vi "Begin.vi"(8 "error in":errorcluster) -> (0 "error out":errorcluster)   [LabVIEW 2020]
doc: "Called before other user functions, this VI is expected to open initial I/O refnums, load in file data, and do all program initialization. Notice that the <B>error out</B> terminal is simply used for data flow. Wiring it to other structures or subVIs ensures that this VI runs first."
uses:
  <vilib>/Rock Robotics/WPI/ThirdParty/Phoenix-LabVIEW/Motor Controller/Controls/CTRE_Phoenix_MotorControl_TalonFXMotorControllerConfigurables.ctl
  <vilib>/Rock Robotics/WPI/ThirdParty/Phoenix-LabVIEW/Motor Controller/Controls/CTRE_Phoenix_MotorControl_BaseConfigurables.ctl
  <vilib>/Rock Robotics/WPI/ThirdParty/Phoenix-LabVIEW/Motor Controller/Controls/CTRE_Phoenix_MotorControl_VelocityMeasurementPeriod.ctl
  <vilib>/Rock Robotics/WPI/ThirdParty/Phoenix-LabVIEW/Motor Controller/Controls/CTRE_Phoenix_MotorControl_SlotStructure.ctl
  <vilib>/Rock Robotics/WPI/ThirdParty/Phoenix-LabVIEW/Motor Controller/Controls/CTRE_Phoenix_MotorControl_FilterStruct.ctl
  <vilib>/Rock Robotics/WPI/ThirdParty/Phoenix-LabVIEW/Motor Controller/Controls/CTRE_Phoenix_MotorControl_RemoteSourceType.ctl
  <vilib>/Rock Robotics/WPI/ThirdParty/Phoenix-LabVIEW/Controls/CTRE_Phoenix_CustomParamConfiguration.ctl
  <vilib>/Rock Robotics/WPI/ThirdParty/Phoenix-LabVIEW/Motor Controller/Controls/CTRE_Phoenix_MotorControl_FeedbackDevice_TalonFX.ctl
  <vilib>/Rock Robotics/WPI/ThirdParty/Phoenix-LabVIEW/Motor Controller/Controls/CTRE_Phoenix_MotorControl_LimitSwitchNormal.ctl
  <vilib>/Rock Robotics/WPI/ThirdParty/Phoenix-LabVIEW/Motor Controller/Controls/CTRE_Phoenix_MotorControl_LimitSwitchSource_Local.ctl
  <vilib>/Rock Robotics/WPI/ThirdParty/Phoenix-LabVIEW/Motor Controller/Controls/CTRE_Phoenix_MotorControl_SupplyCurrentLimitConfiguration.ctl
  <vilib>/Rock Robotics/WPI/ThirdParty/Phoenix-LabVIEW/Motor Controller/Controls/CTRE_Phoenix_MotorControl_StatorCurrentLimitConfiguration.ctl
  <vilib>/Rock Robotics/WPI/ThirdParty/Phoenix-LabVIEW/Motor Controller/Controls/CTRE_Phoenix_MotorControl_MotorCommutation_TalonFX.ctl
  <vilib>/Rock Robotics/WPI/ThirdParty/Phoenix-LabVIEW/CANCoder/Controls/CTRE_Phoenix_CANcoder_AbsoluteSensorRange.ctl
  <vilib>/Rock Robotics/WPI/ThirdParty/Phoenix-LabVIEW/CANCoder/Controls/CTRE_Phoenix_CANcoder_SensorInitializationStrategy.ctl
  <vilib>/Rock Robotics/WPI/ThirdParty/Phoenix-LabVIEW/Motor Controller/Controls/CTRE_Phoenix_MotorControl_NeutralMode.ctl
  <vilib>/Rock Robotics/SystemInterfaces/DIO/FPGA_DIOChannel.ctl
  <vilib>/Rock Robotics/WPI/DriverStation/WPI_DriverStationRobotMode2.ctl
  <vilib>/Rock Robotics/WPI/SafetyOutput/WPI_SafetyOutputConfigMenu.ctl
  <vilib>/Rock Robotics/WPI/RobotDrive/WPI_RobotDriveDevRef.ctl
  <vilib>/Rock Robotics/WPI/MotorControl/WPI_MotorControlDeviceRef.ctl
  <vilib>/Rock Robotics/WPI/MotorControl/WPI_MotorControlType.ctl
  <vilib>/Rock Robotics/SystemInterfaces/DIO/FPGA_DIOPWMChannel.ctl
  <vilib>/Rock Robotics/WPI/PWM/WPI_PWMDeadband.ctl
  <vilib>/Rock Robotics/WPI/ThirdParty/REV Robotics/REVLib/Typedef/Spark MAX Motor Type.ctl
  <vilib>/Rock Robotics/WPI/ThirdParty/REV Robotics/REVLib/Typedef/Spark MAX Idle Mode.ctl
  <vilib>/Rock Robotics/WPI/Joystick/WPI_JoystickDeviceEnum.ctl
  <vilib>/Rock Robotics/Network Tables/NT Write String Array.vi
  Robot Global Data.vi
  <vilib>/Rock Robotics/Network Tables/NT Write Boolean.vi
  <vilib>/Rock Robotics/WPI/Switch/WPI_SwitchOpenCounting.vi
  <vilib>/Rock Robotics/WPI/RobotDrive/WPI_RobotDriveOpen2MotorWithExistingMotors.vi
panel:
  in  "Tab Control":enum32{"DRIVE", "CLIMBING", "SHOOTER"}(tab)=enum."CLIMBING"
  in  "FALCON 500 DRIVE config":T1={"Base Configurables"={"openLoopRamp"=0.0, "closedLoopRamp"=0.0, "peakOutputForward"=1.0, "peakOutputReverse"=-1.0, "nominalOutputForward"=0.0, "nominalOutputReverse"=0.0, "neutralDeadband"=0.04, "voltageCompSaturation"=0.0, "voltageMeasurementFilter"=32, "velocityMeasurementPeriod"=100, "velocityMeasurementWindow"=64, "forwardSoftLimitThreshold"=0, "reverseSoftLimitThreshold"=0, "forwardSoftLimitEnable"=FALSE, "reverseSoftLimitEnable"=FALSE, "slot0"={"P"=0.0, "I"=0.0, "D"=0.0, "F"=0.0, "integralZone"=0.0, "allowableClosedLoopError"=0, "maxIntegralAccumulator"=0.0, "closedLoopPeakOutput"=1.0, "closedLoopPeriod"=1}, "slot1"={"P"=0.0, "I"=0.0, "D"=0.0, "F"=0.0, "integralZone"=0.0, "allowableClosedLoopError"=0, "maxIntegralAccumulator"=0.0, "closedLoopPeakOutput"=1.0, "closedLoopPeriod"=1}, "slot2"={"P"=0.0, "I"=0.0, "D"=0.0, "F"=0.0, "integralZone"=0.0, "allowableClosedLoopError"=0, "maxIntegralAccumulator"=0.0, "closedLoopPeakOutput"=1.0, "closedLoopPeriod"=1}, "slot3"={"P"=0.0, "I"=0.0, "D"=0.0, "F"=0.0, "integralZone"=0.0, "allowableClosedLoopError"=0, "maxIntegralAccumulator"=0.0, "closedLoopPeakOutput"=1.0, "closedLoopPeriod"=1}, "auxPIDPolarity"=FALSE, "remoteFilter0"={"remoteSensorDeviceID"=0, "remoteSensorSource"=enum."Off"}, "remoteFilter1"={"remoteSensorDeviceID"=0, "remoteSensorSource"=enum."Off"}, "motionCruiseVelocity"=0, "motionAcceleration"=0, "motionProfileTrajectoryPeriod"=0, "feedbackNotContinuous"=FALSE, "remoteSensorClosedLoopDisableNeutralOnLOS"=FALSE, "clearPositionOnLimitF"=FALSE, "clearPositionOnLimitR"=FALSE, "clearPositionOnQuadIdx"=FALSE, "limitSwitchDisableNeutralOnLOS"=FALSE, "softLimitDisableNeutralOnLOS"=FALSE, "pulseWidthPeriod_EdgesPerRot"=1, "pulseWidthPeriod_FilterWindowSz"=1, "customParam"={"customParam0"=0, "customParam1"=0}, "trajectoryInterpolationEnable"=TRUE}, "primaryPID"={"selectedFeedbackCoefficient"=1.0, "selectedFeedbackSensor"=1}, "auxiliaryPID"={"selectedFeedbackCoefficient"=1.0, "selectedFeedbackSensor"=1}, "forwardLimitSwitchNormal"=enum."Normally Open", "reverseLimitSwitchNormal"=enum."Normally Open", "forwardLimitSwitchDeviceID"=0, "reverseLimitSwitchDeviceID"=0, "forwardLimitSwitchSource"=enum."Feedback Connector", "reverseLimitSwitchSource"=enum."Feedback Connector", "sum0Term"=1, "sum1Term"=1, "diff0Term"=1, "diff1Term"=1, "Supply Current Limit Configuration"={"Enable?"=FALSE, "Current Limit"=0.0, "Threshold Current"=0.0, "Threshold Time"=0.0}, "Stator Current Limit Configuration"={"Enable?"=FALSE, "Current Limit"=0.0, "Threshold Current"=0.0, "Threshold Time"=0.0}, "Motor Commutation"=enum."Trapezoidal", "Absolute Sensor Range"=enum."Unsigned [0 to 360)", "Integrated Sensor Offset (Degrees)"=0.0, "Sensor Initialization Strategy"=enum."Boot To Zero"} {"diff1Term" items=["Integrated Sensor"=1, "Sensor Sum (S0 + S1)"=9, "Sensor Difference (D0 - D1)"=10, "Remote Source 0"=11, "Remote Source 1"=12, "None"=14, "Software Emulated"=15]; "diff0Term" items=["Integrated Sensor"=1, "Sensor Sum (S0 + S1)"=9, "Sensor Difference (D0 - D1)"=10, "Remote Source 0"=11, "Remote Source 1"=12, "None"=14, "Software Emulated"=15]; "sum1Term" items=["Integrated Sensor"=1, "Sensor Sum (S0 + S1)"=9, "Sensor Difference (D0 - D1)"=10, "Remote Source 0"=11, "Remote Source 1"=12, "None"=14, "Software Emulated"=15]; "sum0Term" items=["Integrated Sensor"=1, "Sensor Sum (S0 + S1)"=9, "Sensor Difference (D0 - D1)"=10, "Remote Source 0"=11, "Remote Source 1"=12, "None"=14, "Software Emulated"=15]; "auxiliaryPID"."selectedFeedbackSensor" items=["Integrated Sensor"=1, "Sensor Sum (S0 + S1)"=9, "Sensor Difference (D0 - D1)"=10, "Remote Source 0"=11, "Remote Source 1"=12, "None"=14, "Software Emulated"=15]; "primaryPID"."selectedFeedbackSensor" items=["Integrated Sensor"=1, "Sensor Sum (S0 + S1)"=9, "Sensor Difference (D0 - D1)"=10, "Remote Source 0"=11, "Remote Source 1"=12, "None"=14, "Software Emulated"=15]; "Base Configurables"."velocityMeasurementPeriod" items=["Period_1ms"=1, "Period_2ms"=2, "Period_5ms"=5, "Period_10ms"=10, "Period_20ms"=20, "Period_25ms"=25, "Period_50ms"=50, "Period_100ms"=100]}
  in  "drive wheel diameter (in)":dbl format="%.3g"
  in  "drive gearbox ratio":dbl
  out "wheel circumference":dbl
  in  "MASTER LEFT DRIVE CAN ID":u8=2
  in  "FALCON Climbing config":T1={"Base Configurables"={"openLoopRamp"=0.0, "closedLoopRamp"=0.0, "peakOutputForward"=1.0, "peakOutputReverse"=-1.0, "nominalOutputForward"=0.0, "nominalOutputReverse"=0.0, "neutralDeadband"=0.04, "voltageCompSaturation"=0.0, "voltageMeasurementFilter"=32, "velocityMeasurementPeriod"=100, "velocityMeasurementWindow"=64, "forwardSoftLimitThreshold"=0, "reverseSoftLimitThreshold"=0, "forwardSoftLimitEnable"=FALSE, "reverseSoftLimitEnable"=FALSE, "slot0"={"P"=0.0, "I"=0.0, "D"=0.0, "F"=0.0, "integralZone"=0.0, "allowableClosedLoopError"=0, "maxIntegralAccumulator"=0.0, "closedLoopPeakOutput"=1.0, "closedLoopPeriod"=1}, "slot1"={"P"=0.0, "I"=0.0, "D"=0.0, "F"=0.0, "integralZone"=0.0, "allowableClosedLoopError"=0, "maxIntegralAccumulator"=0.0, "closedLoopPeakOutput"=1.0, "closedLoopPeriod"=1}, "slot2"={"P"=0.0, "I"=0.0, "D"=0.0, "F"=0.0, "integralZone"=0.0, "allowableClosedLoopError"=0, "maxIntegralAccumulator"=0.0, "closedLoopPeakOutput"=1.0, "closedLoopPeriod"=1}, "slot3"={"P"=0.0, "I"=0.0, "D"=0.0, "F"=0.0, "integralZone"=0.0, "allowableClosedLoopError"=0, "maxIntegralAccumulator"=0.0, "closedLoopPeakOutput"=1.0, "closedLoopPeriod"=1}, "auxPIDPolarity"=FALSE, "remoteFilter0"={"remoteSensorDeviceID"=0, "remoteSensorSource"=enum."Off"}, "remoteFilter1"={"remoteSensorDeviceID"=0, "remoteSensorSource"=enum."Off"}, "motionCruiseVelocity"=0, "motionAcceleration"=0, "motionProfileTrajectoryPeriod"=0, "feedbackNotContinuous"=FALSE, "remoteSensorClosedLoopDisableNeutralOnLOS"=FALSE, "clearPositionOnLimitF"=FALSE, "clearPositionOnLimitR"=FALSE, "clearPositionOnQuadIdx"=FALSE, "limitSwitchDisableNeutralOnLOS"=FALSE, "softLimitDisableNeutralOnLOS"=FALSE, "pulseWidthPeriod_EdgesPerRot"=1, "pulseWidthPeriod_FilterWindowSz"=1, "customParam"={"customParam0"=0, "customParam1"=0}, "trajectoryInterpolationEnable"=TRUE}, "primaryPID"={"selectedFeedbackCoefficient"=1.0, "selectedFeedbackSensor"=1}, "auxiliaryPID"={"selectedFeedbackCoefficient"=1.0, "selectedFeedbackSensor"=1}, "forwardLimitSwitchNormal"=enum."Normally Open", "reverseLimitSwitchNormal"=enum."Normally Open", "forwardLimitSwitchDeviceID"=0, "reverseLimitSwitchDeviceID"=0, "forwardLimitSwitchSource"=enum."Feedback Connector", "reverseLimitSwitchSource"=enum."Feedback Connector", "sum0Term"=1, "sum1Term"=1, "diff0Term"=1, "diff1Term"=1, "Supply Current Limit Configuration"={"Enable?"=FALSE, "Current Limit"=0.0, "Threshold Current"=0.0, "Threshold Time"=0.0}, "Stator Current Limit Configuration"={"Enable?"=FALSE, "Current Limit"=0.0, "Threshold Current"=0.0, "Threshold Time"=0.0}, "Motor Commutation"=enum."Trapezoidal", "Absolute Sensor Range"=enum."Unsigned [0 to 360)", "Integrated Sensor Offset (Degrees)"=0.0, "Sensor Initialization Strategy"=enum."Boot To Zero"} {"diff1Term" items=["Integrated Sensor"=1, "Sensor Sum (S0 + S1)"=9, "Sensor Difference (D0 - D1)"=10, "Remote Source 0"=11, "Remote Source 1"=12, "None"=14, "Software Emulated"=15]; "diff0Term" items=["Integrated Sensor"=1, "Sensor Sum (S0 + S1)"=9, "Sensor Difference (D0 - D1)"=10, "Remote Source 0"=11, "Remote Source 1"=12, "None"=14, "Software Emulated"=15]; "sum1Term" items=["Integrated Sensor"=1, "Sensor Sum (S0 + S1)"=9, "Sensor Difference (D0 - D1)"=10, "Remote Source 0"=11, "Remote Source 1"=12, "None"=14, "Software Emulated"=15]; "sum0Term" items=["Integrated Sensor"=1, "Sensor Sum (S0 + S1)"=9, "Sensor Difference (D0 - D1)"=10, "Remote Source 0"=11, "Remote Source 1"=12, "None"=14, "Software Emulated"=15]; "auxiliaryPID"."selectedFeedbackSensor" items=["Integrated Sensor"=1, "Sensor Sum (S0 + S1)"=9, "Sensor Difference (D0 - D1)"=10, "Remote Source 0"=11, "Remote Source 1"=12, "None"=14, "Software Emulated"=15]; "primaryPID"."selectedFeedbackSensor" items=["Integrated Sensor"=1, "Sensor Sum (S0 + S1)"=9, "Sensor Difference (D0 - D1)"=10, "Remote Source 0"=11, "Remote Source 1"=12, "None"=14, "Software Emulated"=15]; "Base Configurables"."velocityMeasurementPeriod" items=["Period_1ms"=1, "Period_2ms"=2, "Period_5ms"=5, "Period_10ms"=10, "Period_20ms"=20, "Period_25ms"=25, "Period_50ms"=50, "Period_100ms"=100]}
  in  "Motor Control Neutral Mode":T16=enum."Override to Brake"
  in  "CLIMBER LEFT CAN ID":u8=6
  in  "ARM LEFT CAN ID":u8=11
  in  "CLIMBER RIGHT CAN ID":u8=7
  in  "ARM RIGHT CAN ID":u8=15
  in  "FALCON shooter config":T1={"Base Configurables"={"openLoopRamp"=0.0, "closedLoopRamp"=0.0, "peakOutputForward"=1.0, "peakOutputReverse"=-1.0, "nominalOutputForward"=0.0, "nominalOutputReverse"=0.0, "neutralDeadband"=0.04, "voltageCompSaturation"=0.0, "voltageMeasurementFilter"=32, "velocityMeasurementPeriod"=100, "velocityMeasurementWindow"=64, "forwardSoftLimitThreshold"=0, "reverseSoftLimitThreshold"=0, "forwardSoftLimitEnable"=FALSE, "reverseSoftLimitEnable"=FALSE, "slot0"={"P"=0.0, "I"=0.0, "D"=0.0, "F"=0.0, "integralZone"=0.0, "allowableClosedLoopError"=0, "maxIntegralAccumulator"=0.0, "closedLoopPeakOutput"=1.0, "closedLoopPeriod"=1}, "slot1"={"P"=0.0, "I"=0.0, "D"=0.0, "F"=0.0, "integralZone"=0.0, "allowableClosedLoopError"=0, "maxIntegralAccumulator"=0.0, "closedLoopPeakOutput"=1.0, "closedLoopPeriod"=1}, "slot2"={"P"=0.0, "I"=0.0, "D"=0.0, "F"=0.0, "integralZone"=0.0, "allowableClosedLoopError"=0, "maxIntegralAccumulator"=0.0, "closedLoopPeakOutput"=1.0, "closedLoopPeriod"=1}, "slot3"={"P"=0.0, "I"=0.0, "D"=0.0, "F"=0.0, "integralZone"=0.0, "allowableClosedLoopError"=0, "maxIntegralAccumulator"=0.0, "closedLoopPeakOutput"=1.0, "closedLoopPeriod"=1}, "auxPIDPolarity"=FALSE, "remoteFilter0"={"remoteSensorDeviceID"=0, "remoteSensorSource"=enum."Off"}, "remoteFilter1"={"remoteSensorDeviceID"=0, "remoteSensorSource"=enum."Off"}, "motionCruiseVelocity"=0, "motionAcceleration"=0, "motionProfileTrajectoryPeriod"=0, "feedbackNotContinuous"=FALSE, "remoteSensorClosedLoopDisableNeutralOnLOS"=FALSE, "clearPositionOnLimitF"=FALSE, "clearPositionOnLimitR"=FALSE, "clearPositionOnQuadIdx"=FALSE, "limitSwitchDisableNeutralOnLOS"=FALSE, "softLimitDisableNeutralOnLOS"=FALSE, "pulseWidthPeriod_EdgesPerRot"=1, "pulseWidthPeriod_FilterWindowSz"=1, "customParam"={"customParam0"=0, "customParam1"=0}, "trajectoryInterpolationEnable"=TRUE}, "primaryPID"={"selectedFeedbackCoefficient"=1.0, "selectedFeedbackSensor"=1}, "auxiliaryPID"={"selectedFeedbackCoefficient"=1.0, "selectedFeedbackSensor"=1}, "forwardLimitSwitchNormal"=enum."Normally Open", "reverseLimitSwitchNormal"=enum."Normally Open", "forwardLimitSwitchDeviceID"=0, "reverseLimitSwitchDeviceID"=0, "forwardLimitSwitchSource"=enum."Feedback Connector", "reverseLimitSwitchSource"=enum."Feedback Connector", "sum0Term"=1, "sum1Term"=1, "diff0Term"=1, "diff1Term"=1, "Supply Current Limit Configuration"={"Enable?"=FALSE, "Current Limit"=0.0, "Threshold Current"=0.0, "Threshold Time"=0.0}, "Stator Current Limit Configuration"={"Enable?"=FALSE, "Current Limit"=0.0, "Threshold Current"=0.0, "Threshold Time"=0.0}, "Motor Commutation"=enum."Trapezoidal", "Absolute Sensor Range"=enum."Unsigned [0 to 360)", "Integrated Sensor Offset (Degrees)"=0.0, "Sensor Initialization Strategy"=enum."Boot To Zero"} {"diff1Term" items=["Integrated Sensor"=1, "Sensor Sum (S0 + S1)"=9, "Sensor Difference (D0 - D1)"=10, "Remote Source 0"=11, "Remote Source 1"=12, "None"=14, "Software Emulated"=15]; "diff0Term" items=["Integrated Sensor"=1, "Sensor Sum (S0 + S1)"=9, "Sensor Difference (D0 - D1)"=10, "Remote Source 0"=11, "Remote Source 1"=12, "None"=14, "Software Emulated"=15]; "sum1Term" items=["Integrated Sensor"=1, "Sensor Sum (S0 + S1)"=9, "Sensor Difference (D0 - D1)"=10, "Remote Source 0"=11, "Remote Source 1"=12, "None"=14, "Software Emulated"=15]; "sum0Term" items=["Integrated Sensor"=1, "Sensor Sum (S0 + S1)"=9, "Sensor Difference (D0 - D1)"=10, "Remote Source 0"=11, "Remote Source 1"=12, "None"=14, "Software Emulated"=15]; "auxiliaryPID"."selectedFeedbackSensor" items=["Integrated Sensor"=1, "Sensor Sum (S0 + S1)"=9, "Sensor Difference (D0 - D1)"=10, "Remote Source 0"=11, "Remote Source 1"=12, "None"=14, "Software Emulated"=15]; "primaryPID"."selectedFeedbackSensor" items=["Integrated Sensor"=1, "Sensor Sum (S0 + S1)"=9, "Sensor Difference (D0 - D1)"=10, "Remote Source 0"=11, "Remote Source 1"=12, "None"=14, "Software Emulated"=15]; "Base Configurables"."velocityMeasurementPeriod" items=["Period_1ms"=1, "Period_2ms"=2, "Period_5ms"=5, "Period_10ms"=10, "Period_20ms"=20, "Period_25ms"=25, "Period_50ms"=50, "Period_100ms"=100]}
  in  "Motor Control Neutral Mode 2":T16=enum."Override to Brake"
  in  "SHOOTER CAN ID":u8=8
  in  "KICKER CAN ID":u8=10
  in  "KICKER COUNT DIO":T17
  # "Sum and Diff terms are ways to select more than one sensor as a feedback device. \n Sum 0 is the first feedback device to be used for the Sum term.\n Sum 1 is the feedback device to be added to Sum 0 for the Sum term.\n Diff 0 and Diff 1 work in a similar manner."
  # "These are only applicable\nif using a remote limit switch.\n\nLocal limit switches/no limit\nswitches do not use this."
  # "Current is below Current Limit AND\n\n(Requested output is weaker** than applied motor\noutput OR is in the opposite direction).\n/\nMotor output is set to requested output."
  # "Current is above Threshold Current for Threshold Time\n/\nReduce motor output (towards neutral)."
  # "Current is below Current Limit.\n/\nRamp motor output towards requested output."
  # "Current is above Current Limit.\n/\nReduce motor output (towards neutral)."
  # "*If the configured Peak Threshold is less than the Continuous Threshold, the applied Peak Threshold is set equal to the Configured Continuous Threshold in firmware.\n** Both requested output and applied motor output are in the same direction, and requested output is closer to neutral."
  # "False: Primary Output = PID[0] + PID[1]  ---  Auxiliary Output = PID[0] - PID[1]\nTrue:  Primary Output = PID[0] - PID[1] --- Auxiliary Output = PID[0] + PID[1]"
  # "Enable the motion profile executor to perform linear interpolation between profile points.  Defaults to True."
  # "Sum and Diff terms are ways to select more than one sensor as a feedback device. \n Sum 0 is the first feedback device to be used for the Sum term.\n Sum 1 is the feedback device to be added to Sum 0 for the Sum term.\n Diff 0 and Diff 1 work in a similar manner."
  # "These are only applicable\nif using a remote limit switch.\n\nLocal limit switches/no limit\nswitches do not use this."
  # "Current is below Current Limit AND\n\n(Requested output is weaker** than applied motor\noutput OR is in the opposite direction).\n/\nMotor output is set to requested output."
  # "Current is above Threshold Current for Threshold Time\n/\nReduce motor output (towards neutral)."
  # "Current is below Current Limit.\n/\nRamp motor output towards requested output."
  # "Current is above Current Limit.\n/\nReduce motor output (towards neutral)."
  # "*If the configured Peak Threshold is less than the Continuous Threshold, the applied Peak Threshold is set equal to the Configured Continuous Threshold in firmware.\n** Both requested output and applied motor output are in the same direction, and requested output is closer to neutral."
  # "False: Primary Output = PID[0] + PID[1]  ---  Auxiliary Output = PID[0] - PID[1]\nTrue:  Primary Output = PID[0] - PID[1] --- Auxiliary Output = PID[0] + PID[1]"
  # "Enable the motion profile executor to perform linear interpolation between profile points.  Defaults to True."
  # "Sum and Diff terms are ways to select more than one sensor as a feedback device. \n Sum 0 is the first feedback device to be used for the Sum term.\n Sum 1 is the feedback device to be added to Sum 0 for the Sum term.\n Diff 0 and Diff 1 work in a similar manner."
  # "These are only applicable\nif using a remote limit switch.\n\nLocal limit switches/no limit\nswitches do not use this."
  # "Current is below Current Limit AND\n\n(Requested output is weaker** than applied motor\noutput OR is in the opposite direction).\n/\nMotor output is set to requested output."
  # "Current is above Threshold Current for Threshold Time\n/\nReduce motor output (towards neutral)."
  # "Current is below Current Limit.\n/\nRamp motor output towards requested output."
  # "Current is above Current Limit.\n/\nReduce motor output (towards neutral)."
  # "*If the configured Peak Threshold is less than the Continuous Threshold, the applied Peak Threshold is set equal to the Configured Continuous Threshold in firmware.\n** Both requested output and applied motor output are in the same direction, and requested output is closer to neutral."
  # "False: Primary Output = PID[0] + PID[1]  ---  Auxiliary Output = PID[0] - PID[1]\nTrue:  Primary Output = PID[0] - PID[1] --- Auxiliary Output = PID[0] + PID[1]"
  # "Enable the motion profile executor to perform linear interpolation between profile points.  Defaults to True."
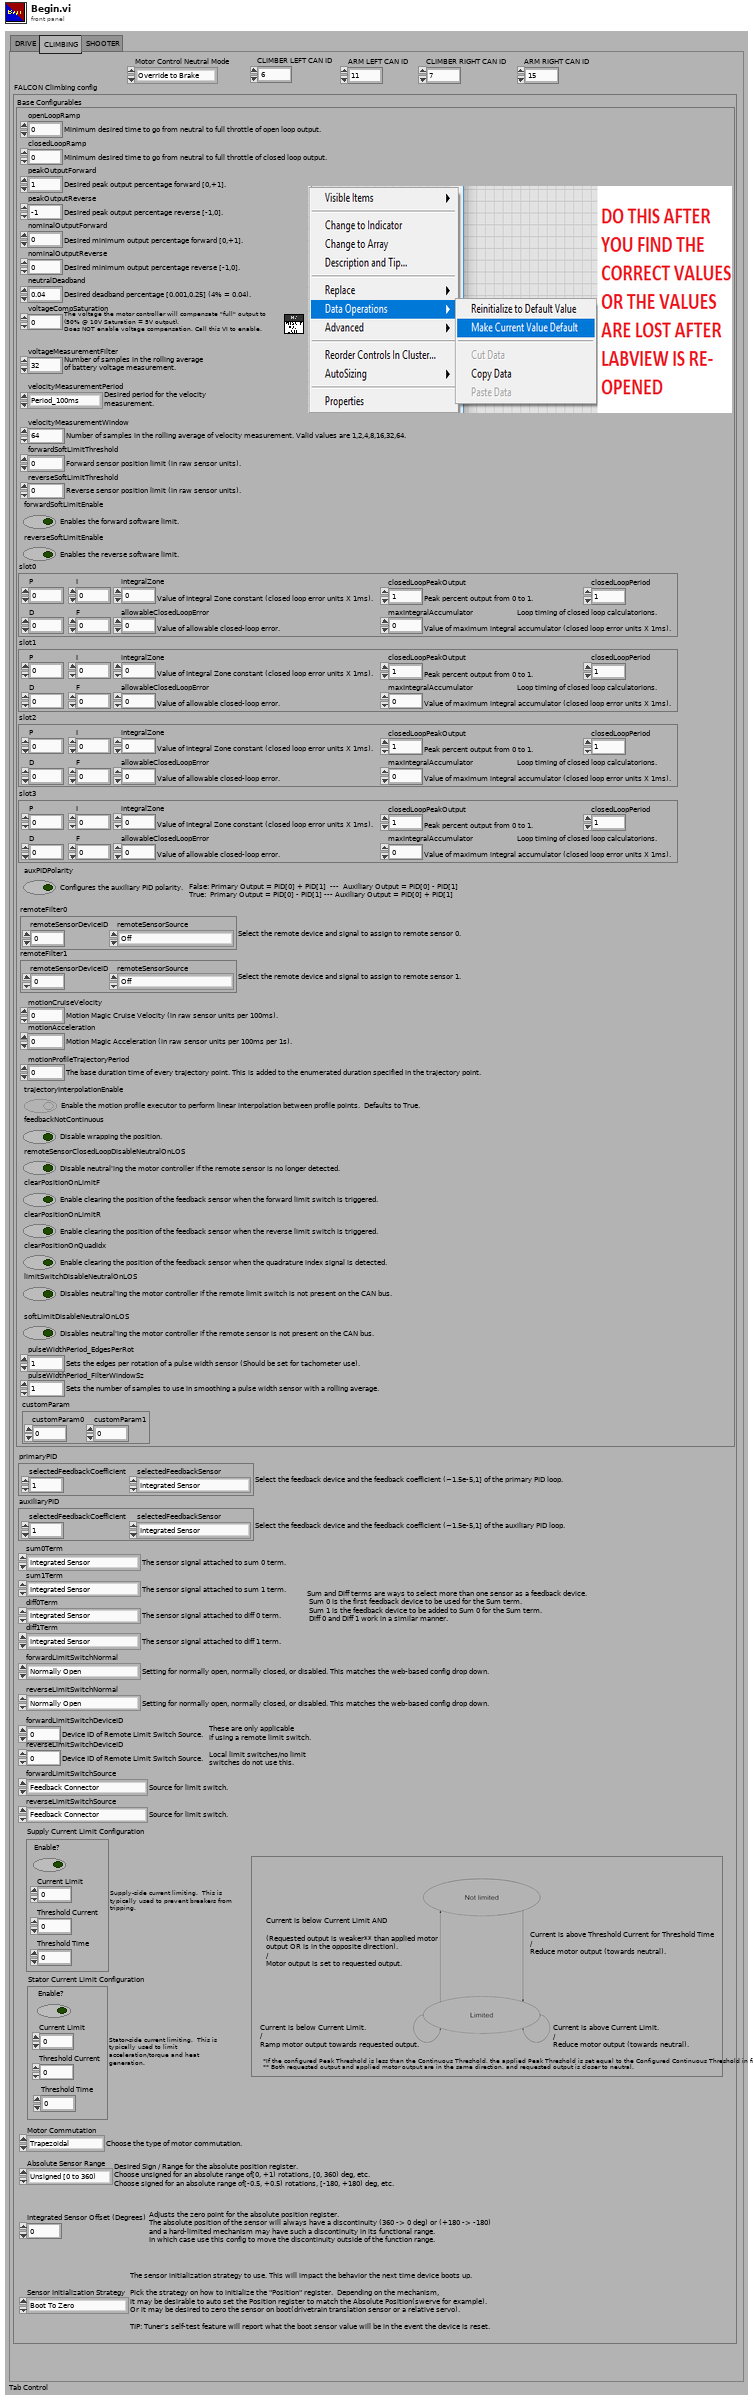
[diagram p1: front panel]
types:
  T1 = typedef "CTRE_Phoenix_MotorControl_TalonFXMotorControllerConfigurables.ctl" = cluster{"Base Configurables":T2, "primaryPID":cluster{"selectedFeedbackCoefficient":dbl, "selectedFeedbackSensor":T8}, "auxiliaryPID":cluster{"selectedFeedbackCoefficient":dbl, "selectedFeedbackSensor":T8}, "forwardLimitSwitchNormal":T9, "reverseLimitSwitchNormal":T9, "forwardLimitSwitchDeviceID":i32, "reverseLimitSwitchDeviceID":i32, "forwardLimitSwitchSource":T10, "reverseLimitSwitchSource":T10, "sum0Term":T8, "sum1Term":T8, "diff0Term":T8, "diff1Term":T8, "Supply Current Limit Configuration":T11, "Stator Current Limit Configuration":T12, "Motor Commutation":T13, "Absolute Sensor Range":T14, "Integrated Sensor Offset (Degrees)":dbl, "Sensor Initialization Strategy":T15}
  T2 = typedef "CTRE_Phoenix_MotorControl_BaseConfigurables.ctl" = cluster{"openLoopRamp":dbl, "closedLoopRamp":dbl, "peakOutputForward":dbl, "peakOutputReverse":dbl, "nominalOutputForward":dbl, "nominalOutputReverse":dbl, "neutralDeadband":dbl, "voltageCompSaturation":dbl, "voltageMeasurementFilter":i32, "velocityMeasurementPeriod":T3, "velocityMeasurementWindow":i32, "forwardSoftLimitThreshold":i32, "reverseSoftLimitThreshold":i32, "forwardSoftLimitEnable":bool, "reverseSoftLimitEnable":bool, "slot0":T4, "slot1":T4, "slot2":T4, "slot3":T4, "auxPIDPolarity":bool, "remoteFilter0":T5, "remoteFilter1":T5, "motionCruiseVelocity":i32, "motionAcceleration":i32, "motionProfileTrajectoryPeriod":i32, "feedbackNotContinuous":bool, "remoteSensorClosedLoopDisableNeutralOnLOS":bool, "clearPositionOnLimitF":bool, "clearPositionOnLimitR":bool, "clearPositionOnQuadIdx":bool, "limitSwitchDisableNeutralOnLOS":bool, "softLimitDisableNeutralOnLOS":bool, "pulseWidthPeriod_EdgesPerRot":i32, "pulseWidthPeriod_FilterWindowSz":i32, "customParam":T7, "trajectoryInterpolationEnable":bool}
  T3 = typedef "CTRE_Phoenix_MotorControl_VelocityMeasurementPeriod.ctl" = u16
  T4 = typedef "CTRE_Phoenix_MotorControl_SlotStructure.ctl" = cluster{"P":dbl, "I":dbl, "D":dbl, "F":dbl, "integralZone":dbl, "allowableClosedLoopError":i32, "maxIntegralAccumulator":dbl, "closedLoopPeakOutput":dbl, "closedLoopPeriod":i32}
  T5 = typedef "CTRE_Phoenix_MotorControl_FilterStruct.ctl" = cluster{"remoteSensorDeviceID":u8, "remoteSensorSource":T6}
  T6 = typedef "CTRE_Phoenix_MotorControl_RemoteSourceType.ctl" = enum16{"Off", "Talon SRX Selected Sensor", "Pigeon IMU Yaw", "Pigeon IMU Pitch", "Pigeon IMU Roll", "CANifier Quadrature", "CANifier PWM Input 0", "CANifier PWM Input 1", "CANifier PWM Input 2", "CANifier PWM Input 3", "Gadgeteer Pigeon Yaw", "Gadgeteer Pigeon Pitch", "Gadgeteer Pigeon Roll", "CANCoder"}
  T7 = typedef "CTRE_Phoenix_CustomParamConfiguration.ctl" = cluster{"customParam0":i32, "customParam1":i32}
  T8 = typedef "CTRE_Phoenix_MotorControl_FeedbackDevice_TalonFX.ctl" = i8
  T9 = typedef "CTRE_Phoenix_MotorControl_LimitSwitchNormal.ctl" = enum16{"Normally Open", "Normally Closed", "Disabled"}
  T10 = typedef "CTRE_Phoenix_MotorControl_LimitSwitchSource_Local.ctl" = enum16{"Feedback Connector", "Remote Talon SRX", "Remote CANifier", "Deactivated"}
  T11 = typedef "CTRE_Phoenix_MotorControl_SupplyCurrentLimitConfiguration.ctl" = cluster{"Enable?":bool, "Current Limit":dbl, "Threshold Current":dbl, "Threshold Time":dbl}
  T12 = typedef "CTRE_Phoenix_MotorControl_StatorCurrentLimitConfiguration.ctl" = cluster{"Enable?":bool, "Current Limit":dbl, "Threshold Current":dbl, "Threshold Time":dbl}
  T13 = typedef "CTRE_Phoenix_MotorControl_MotorCommutation_TalonFX.ctl" = enum16{"Trapezoidal"}
  T14 = typedef "CTRE_Phoenix_CANcoder_AbsoluteSensorRange.ctl" = enum16{"Unsigned [0 to 360)", "Signed [-180 to +180)"}
  T15 = typedef "CTRE_Phoenix_CANcoder_SensorInitializationStrategy.ctl" = enum16{"Boot To Zero", "Boot To Absolute Position"}
  T16 = typedef "CTRE_Phoenix_MotorControl_NeutralMode.ctl" = enum8{"EEPROMSetting", "Override to Coast", "Override to Brake"}
  T17 = typedef "FPGA_DIOChannel.ctl" = enum8{"DIO 0", "DIO 1", "DIO 2", "DIO 3", "DIO 4", "DIO 5", "DIO 6", "DIO 7", "DIO 8", "DIO 9", "DIO MXP 0", "DIO MXP 1", "DIO MXP 2", "DIO MXP 3", "DIO MXP 4", "DIO MXP 5", "DIO MXP 6", "DIO MXP 7", "DIO MXP 8", "DIO MXP 9", "DIO MXP 10", "DIO MXP 11", "DIO MXP 12", "DIO MXP 13", "DIO MXP 14", "DIO MXP 15", "SPI Port CS1", "SPI Port CS2", "SPI Port CS3", "SPI Port MISO", "SPI Port MOSI", "Invalid"}
  T18 = typedef "WPI_DriverStationRobotMode2.ctl" = enum16{"Autonomous Disabled", "Autonomous Enabled", "Teleop Disabled", "Teleop Enabled", "Disconnected", "Finish", "Test Disabled", "Test Enabled", "Emergency Stopped"}
  T19 = typedef "WPI_RobotDriveDevRef.ctl" = cluster{"DevStatus":errorcluster, "Motors[]":T20[], "Square Inputs":bool, "Max Output":dbl}
  T20 = typedef "WPI_MotorControlDeviceRef.ctl" = cluster{"DeviceStatus":errorcluster, "Type":T21, "PWM":cluster{"PWM Channel":T22, "DeadBand":T23}, "CAN":cluster{"Device Number":u8, "SetOutput VI Ref":variant, "GetOutput VI Ref":variant, "Enable VI Ref":variant, "Disable VI Ref":variant, "Data":variant}, "Invert":bool, "DIO PWM":cluster{"PWM \"Enable\" Channel":T22, "DIOChannel":T17, "PWM Rate":dbl}}
  T21 = typedef "WPI_MotorControlType.ctl" = enum16{"PWM", "CAN", "DIO PWM"}
  T22 = typedef "FPGA_DIOPWMChannel.ctl" = enum8{"PWM 0", "PWM 1", "PWM 2", "PWM 3", "PWM 4", "PWM 5", "PWM 6", "PWM 7", "PWM 8", "PWM 9", "PWM MXP 0", "PWM MXP 1", "PWM MXP 2", "PWM MXP 3", "PWM MXP 4", "PWM MXP 5", "PWM MXP 6", "PWM MXP 7", "PWM MXP 8", "PWM MXP 9", "Invalid"}
  T23 = typedef "WPI_PWMDeadband.ctl" = cluster{"Name":string, "maxPositivePwm":i32, "minPositivePwm":i32, "centerPwm":i32, "maxNegativePwm":i32, "minNegativePwm":i32, "angularRange":u16}
  T24 = typedef "WPI_SafetyOutputConfigMenu.ctl" = enum16{"Enable", "Disable"}
  T25 = enum16{"FollowerType_PercentOutput", "FollowerType_AuxOutput1"}
  T26 = typedef "Spark MAX Idle Mode.ctl" = enum16{"Coast", "Brake"}
  T27 = typedef "Spark MAX Motor Type.ctl" = enum16{"Brushed", "Brushless"}
  T28 = typedef "WPI_SwitchDevRef.ctl" = cluster{"DevStatus":errorcluster, "DIO Channel":T17, "CntIndex":T29, "Normally Closed":bool}
  T29 = typedef "FPGA_CounterCtrSystemIndex.ctl" = enum8{"Ctr 0", "Ctr 1", "Ctr 2", "Ctr 3", "Ctr 4", "Ctr 5", "Ctr 6", "Ctr 7", "Invalid"}
  T30 = typedef "WPI_JoystickDeviceEnum.ctl" = enum16{"USB 0", "USB 1", "USB 2", "USB 3", "USB 4", "USB 5"}
  T31 = typedef "WPI_JoystickDevRef.ctl" = cluster{"Device":T30}
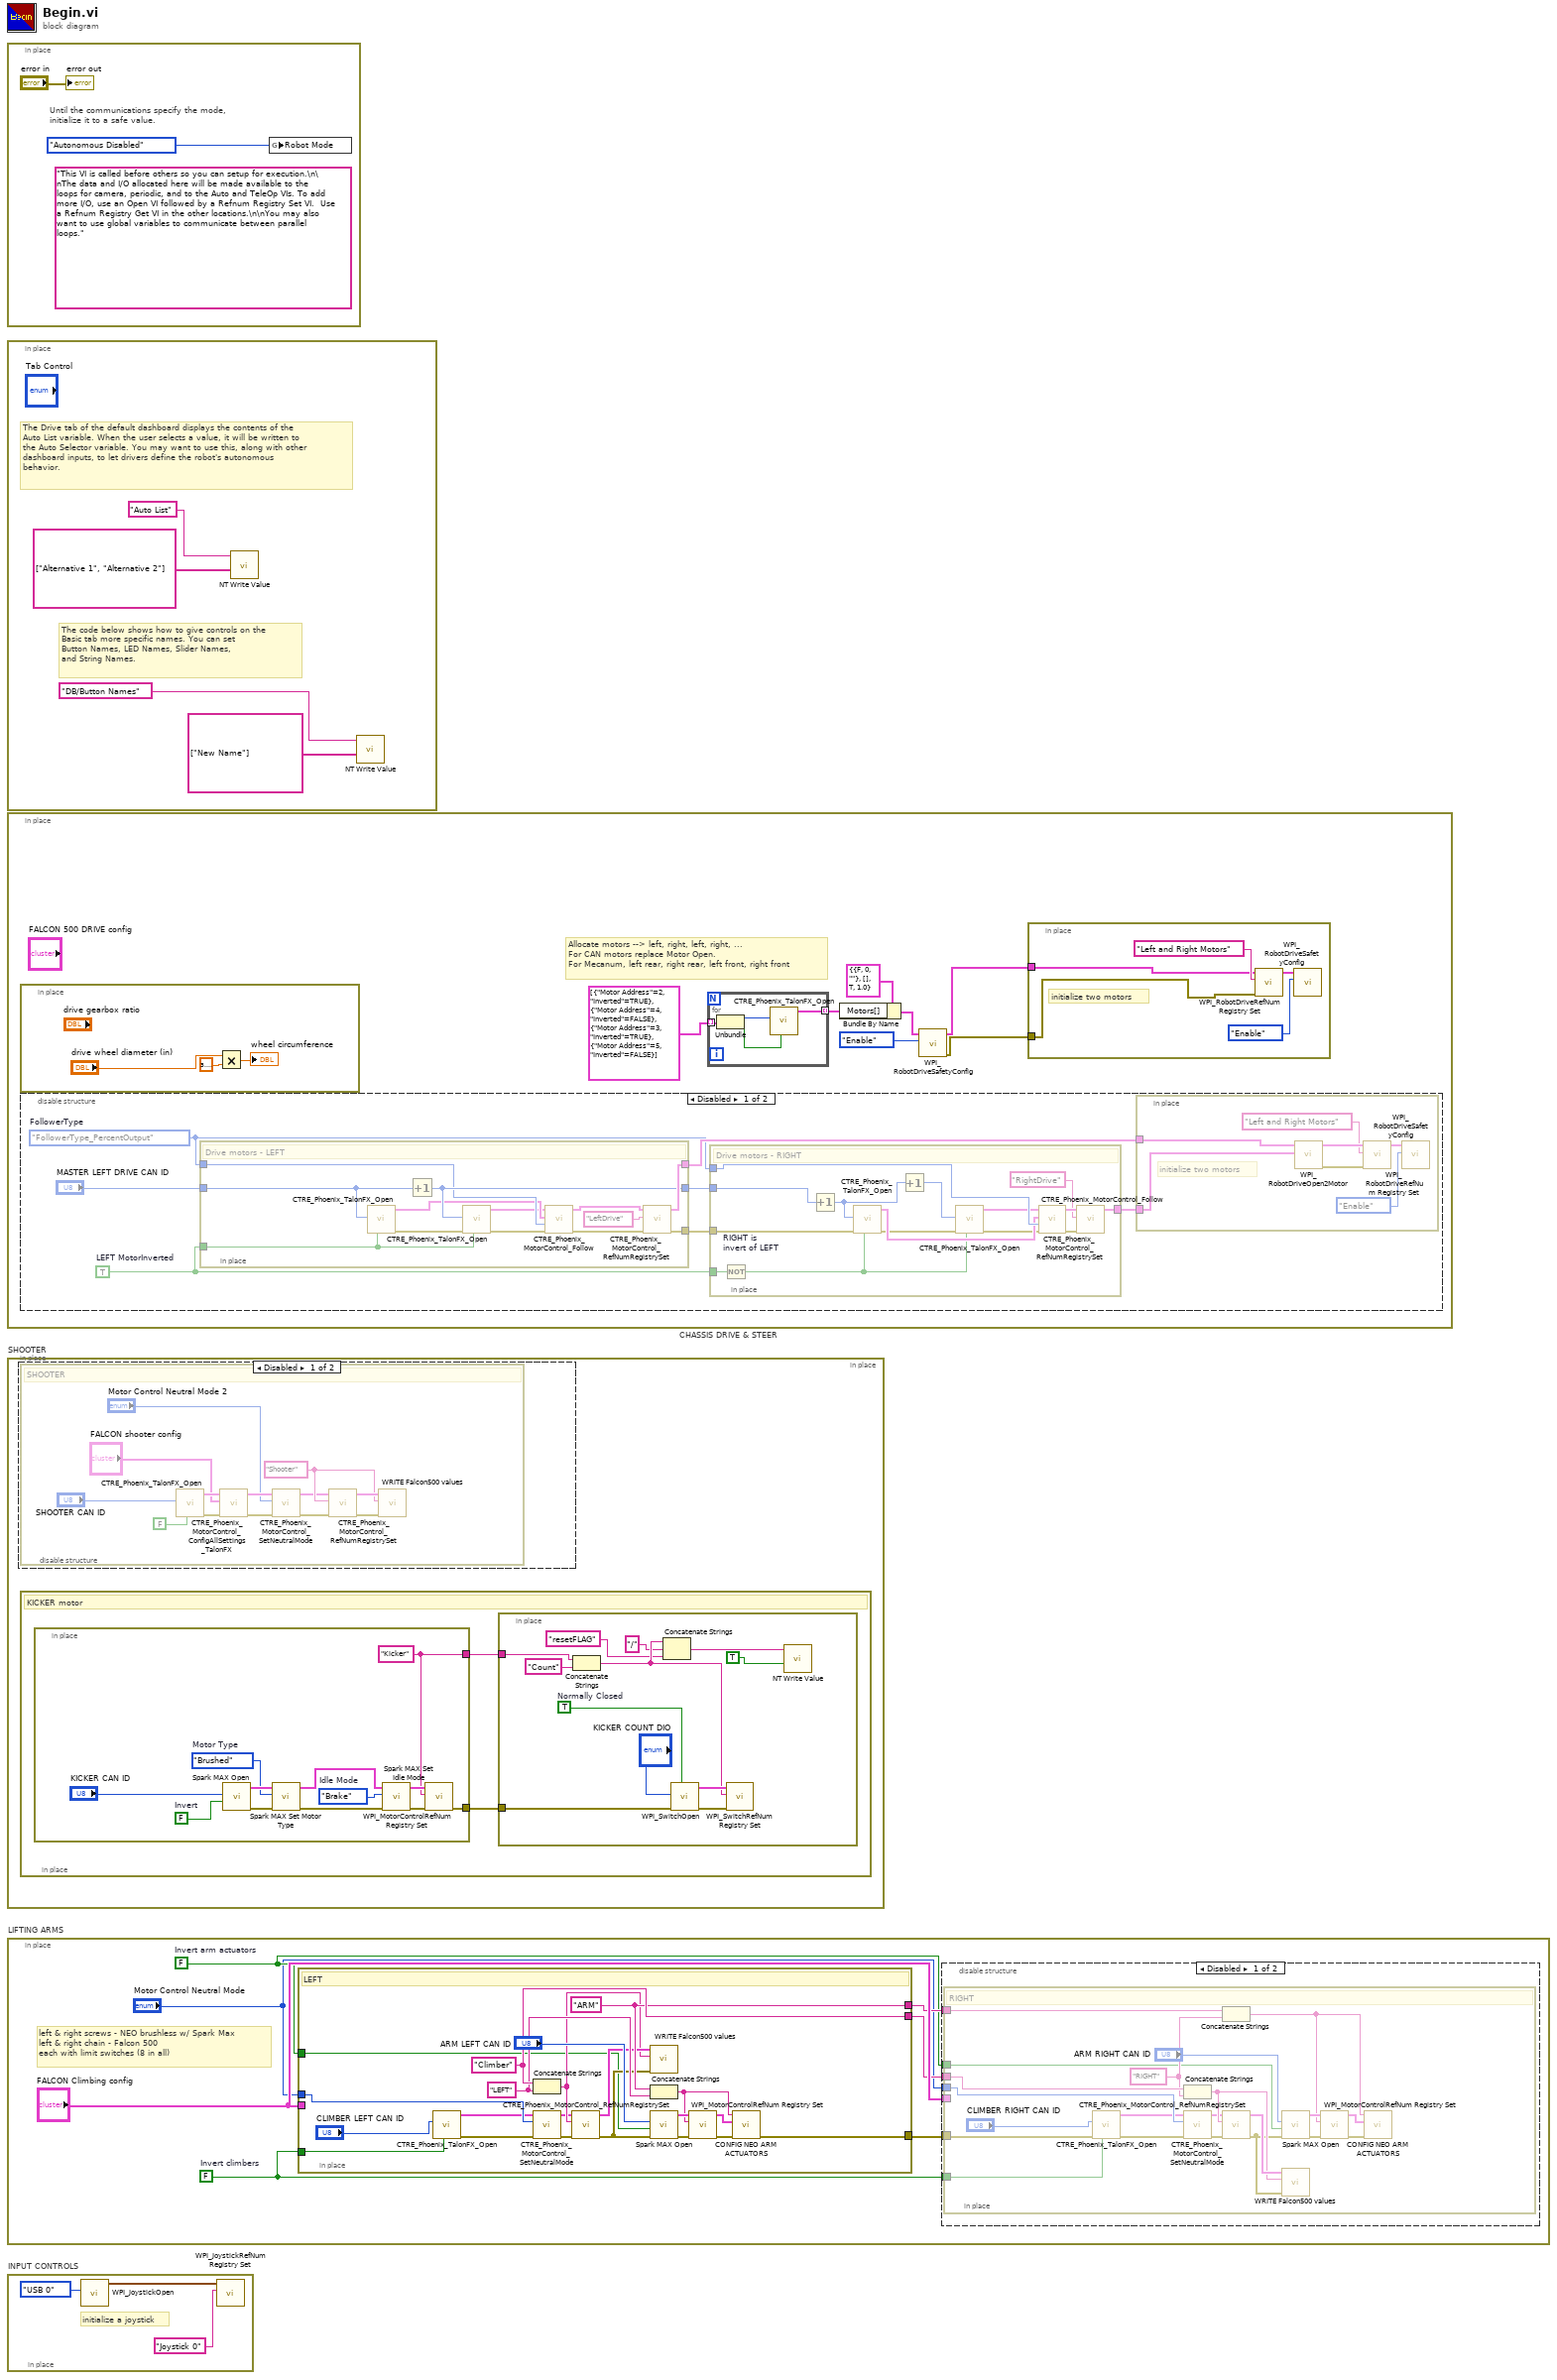
[diagram p0: block diagram]
diagram:
  n1 = in-place {
    (unwired) "This VI is called before others so you can setup for execution.\n\nThe data and I/O allocated here will be made available to the loops for camera, periodic, and to the Auto and TeleOp VIs. To add more I/O, use an Open VI followed by a Refnum Registry Set VI.  Use a Refnum Registry Get VI in the other locations.\n\nYou may also want to use global variables to communicate between parallel loops."
    # "Until the communications specify the mode,\ninitialize it to a safe value."
    n2 = global write "Robot Global Data.vi" "Robot Mode"(WPI_DriverStationRobotMode2."Autonomous Disabled" ("Robot Mode")) -> ()
    "error out" <- "error in"
  }
  n3 = in-place {
    # "The Drive tab of the default dashboard displays the contents of the\nAuto List variable. When the user selects a value, it will be written to\nthe Auto Selector variable. You may want to use this, along with other\ndashboard inputs, to let drivers define the robot's autonomous\nbehavior."
    # "The code below shows how to give controls on the\nBasic tab more specific names. You can set\nButton Names, LED Names, Slider Names,\nand String Names."
    n4 = call-poly <vilib>:"NT Write Value.vi"("String Array"=string[] ["Alternative 1", "Alternative 2"], "Name"="Auto List") -> ()  [unwired: 9 in, 1 out]
    n5 = call-poly <vilib>:"NT Write Value.vi"("String Array"=string[] ["New Name"], "Name"="DB/Button Names") -> ()  [unwired: 9 in, 1 out]
  }
  n6 = in-place "CHASSIS DRIVE & STEER" {
    # "Allocate motors --> left, right, left, right, ... \nFor CAN motors replace Motor Open.\nFor Mecanum, left rear, right rear, left front, right front"
    n7 = in-place {
      n8 = Multiply(x="drive wheel diameter (in)", y=3.141592653589793) -> (x*y=→"wheel circumference":dbl)
    }
    n9 = disable-structure shown="Disabled" {
      frame Disabled {
        w24 = TRUE  # LEFT MotorInverted
        w26 = T25."FollowerType_PercentOutput"  # FollowerType
        n10 = in-place {
          in-place-border: [w56] -> w28
          in-place-border: [w53] -> w29
          in-place-border: w26 -> [w52]
          in-place-border: "MASTER LEFT DRIVE CAN ID" -> [w51]
          in-place-border: w24 -> [w45]
          in-place-border: [w50] -> w23
          # "Drive motors - LEFT"
          n11 = call <vilib>:"CTRE_Phoenix_TalonFX_Open.vi"("Invert"=w45, "Device Number"=w51) -> ("error out"=w48:errorcluster, "PhoenixMotorControlDevRef"=w49:T20)  [unwired: 8 in]
          n12 = Increment(x=w51) -> (x+1=w53:u8)
          n13 = call <vilib>:"CTRE_Phoenix_TalonFX_Open.vi"("Invert"=w45, "error in"=w48, "Device Number"=w53) -> ("error out"=w46:errorcluster, "PhoenixMotorControlDevRef"=w47:T20)  [unwired: 7 in]
          n14 = call <vilib>:"CTRE_Phoenix_MotorControl_Follow.vi"("error in (no error)"=w46, "FollowerType"=w52, "Master Controller to Follow"=w49, "PhoenixMotorControlDevRef"=w47) -> ("error out"=w55:errorcluster, "PhoenixMotorControlDevRef"=w57:T20)  [unwired: 6 in]
          n15 = call <vilib>:"CTRE_Phoenix_MotorControl_RefNumRegistrySet.vi"("error in (no error)"=w55, "refnum name"="LeftDrive", "PhoenixMotorControlDevRef"=w57) -> ("error out"=w50:errorcluster, "PhoenixMotorControlDevRef"=w56:T20)  [unwired: 7 in]
        }
        n16 = in-place {
          in-place-border: [w42] -> w27
          in-place-border: w24 -> [w39]
          in-place-border: w29 -> [w38]
          in-place-border: w26 -> [w36]
          in-place-border: w23 -> [w35]
          # "Drive motors - RIGHT"
          n17 = Not "RIGHT is\ninvert of LEFT"(x=w39) -> (.not. x?=w30:bool)
          n18 = Increment(x=w38) -> (x+1=w37:u8)
          n19 = call <vilib>:"CTRE_Phoenix_TalonFX_Open.vi"("Invert"=w30, "error in"=w35, "Device Number"=w37) -> ("error out"=w33:errorcluster, "PhoenixMotorControlDevRef"=w34:T20)  [unwired: 7 in]
          n20 = Increment(x=w37) -> (x+1=w44:u8)
          n21 = call <vilib>:"CTRE_Phoenix_TalonFX_Open.vi"("Invert"=w30, "error in"=w33, "Device Number"=w44) -> ("error out"=w31:errorcluster, "PhoenixMotorControlDevRef"=w32:T20)  [unwired: 7 in]
          n22 = call <vilib>:"CTRE_Phoenix_MotorControl_Follow.vi"("error in (no error)"=w31, "FollowerType"=w36, "Master Controller to Follow"=w34, "PhoenixMotorControlDevRef"=w32) -> ("error out"=w41:errorcluster, "PhoenixMotorControlDevRef"=w43:T20)  [unwired: 6 in]
          n23 = call <vilib>:"CTRE_Phoenix_MotorControl_RefNumRegistrySet.vi"("error in (no error)"=w41, "refnum name"="RightDrive", "PhoenixMotorControlDevRef"=w43) -> ("PhoenixMotorControlDevRef"=w42:T20)  [unwired: 7 in, 1 out]
        }
        n24 = in-place {
          in-place-border: w28 -> [w59]
          in-place-border: w27 -> [w58]
          # "initialize two motors"
          n25 = call-poly <vilib>:"WPI_RobotDriveOpen2Motor.vi"("Right Motor Dev Ref"=w58, "Left Motor Dev Ref"=w59) -> ("error out"=w62:errorcluster, "RobotDriveDevRef"=w64:T19)  [unwired: 3 in, 5 out]
          n26 = call <vilib>:"WPI_RobotDriveRefNum Registry Set.vi"("error in (no error)"=w62, "refnum name"="Left and Right Motors", "RobotDriveDevRef"=w64) -> ("RobotDriveDevRef"=w61:T19)  [unwired: 1 in, 7 out]
          n27 = call <vilib>:"WPI_RobotDriveSafetyConfig.vi"("mode"=WPI_SafetyOutputConfigMenu."Enable", "RobotDriveDevRef"=w61) -> ()  [unwired: 8 in, 2 out]
        }
      }
      frame Enabled {
      }
    }
    n28 = for {
      tunnel: cluster{"Motor Address":i32, "Inverted":bool}[] [{"Motor Address"=2, "Inverted"=TRUE}, {"Motor Address"=4, "Inverted"=FALSE}, {"Motor Address"=3, "Inverted"=TRUE}, {"Motor Address"=5, "Inverted"=FALSE}] ("Array") -> [w22] mode=indexing
      tunnel: [w19] -> w13 mode=indexing
      n29 = Unbundle(w22) -> ("Motor Address"=w21:i32, "Inverted"=w20:bool)
      n30 = call <vilib>:"CTRE_Phoenix_TalonFX_Open.vi"("Invert"=w20, "Device Number"=w21) -> ("PhoenixMotorControlDevRef"=w19:T20)  [unwired: 8 in, 1 out]
    }
    n31 = Bundle By Name(cluster=T19 {"DevStatus"={"status"=FALSE, "code"=0, "source"=""}, "Motors[]"=[], "Square Inputs"=TRUE, "Max Output"=1.0} ("RobotDriveDevRef"), "Motors[]"=w13) -> (w11:T19)
    n32 = call <vilib>:"WPI_RobotDriveSafetyConfig.vi"("mode"=WPI_SafetyOutputConfigMenu."Enable", "RobotDriveDevRef"=w11) -> ("error out"=w7:errorcluster, "RobotDriveDevRef"=w8:T19)  [unwired: 2 in, 6 out]
    n33 = in-place {
      in-place-border: w8 -> [w15]
      in-place-border: w7 -> [w14]
      # "initialize two motors"
      n34 = call <vilib>:"WPI_RobotDriveRefNum Registry Set.vi"("error in (no error)"=w14, "refnum name"="Left and Right Motors", "RobotDriveDevRef"=w15) -> ("RobotDriveDevRef"=w17:T19)  [unwired: 1 in, 7 out]
      n35 = call <vilib>:"WPI_RobotDriveSafetyConfig.vi"("mode"=WPI_SafetyOutputConfigMenu."Enable", "RobotDriveDevRef"=w17) -> ()  [unwired: 8 in, 2 out]
    }
  }
  n36 = in-place "SHOOTER" {
    n37 = disable-structure shown="Disabled" {
      frame Disabled {
        n38 = in-place {
          w73 = "Shooter" ("refnum name")
          # "SHOOTER"
          n39 = call <vilib>:"CTRE_Phoenix_TalonFX_Open.vi"("Invert"=FALSE, "Device Number"="SHOOTER CAN ID") -> ("error out"=w80:errorcluster, "PhoenixMotorControlDevRef"=w79:T20)  [unwired: 8 in]
          n40 = call <vilib>:"CTRE_Phoenix_MotorControl_ConfigAllSettings_TalonFX.vi"("error in (no error)"=w80, "Talon FX Configurables"="FALCON shooter config", "PhoenixMotorControlDevRef"=w79) -> ("error out"=w69:errorcluster, "PhoenixMotorControlDevRef"=w72:T20)  [unwired: 7 in]
          n41 = call <vilib>:"CTRE_Phoenix_MotorControl_SetNeutralMode.vi"("error in (no error)"=w69, "Motor Control Neutral Mode"="Motor Control Neutral Mode 2", "PhoenixMotorControlDevRef"=w72) -> ("error out"=w70:errorcluster, "PhoenixMotorControlDevRef"=w71:T20)  [unwired: 7 in]
          n42 = call <vilib>:"CTRE_Phoenix_MotorControl_RefNumRegistrySet.vi"("error in (no error)"=w70, "refnum name"=w73, "PhoenixMotorControlDevRef"=w71) -> ("error out"=w74:errorcluster, "PhoenixMotorControlDevRef"=w75:T20)  [unwired: 7 in]
          n43 = call "WRITE Falcon500 values.vi"("PhoenixMotorControlDevRef"=w75, "refnum name"=w73, "error in (no error)"=w74) -> ()  [unwired: 5 in, 2 out]
        }
      }
      frame Enabled {
      }
    }
    n44 = in-place {
      # "KICKER motor"
      n45 = in-place {
        in-place-border: [w85] -> w82
        in-place-border: [w84] -> w81
        w83 = FALSE  # Invert
        w84 = "Kicker" ("refnum name")
        w88 = Spark_MAX_Idle_Mode."Brake"  # Idle Mode
        w91 = Spark_MAX_Motor_Type."Brushed"  # Motor Type
        n46 = call <vilib>:"Spark MAX Open.vi"("Invert"=w83, "Device Number"="KICKER CAN ID") -> ("error out"=w93:errorcluster, "MotorControlDeviceRef"=w92:T20)  [unwired: 8 in]
        n47 = call <vilib>:"Spark MAX Set Motor Type.vi"("error in (no error)"=w93, "Motor Type"=w91, "MotorControlDevRef"=w92) -> ("error out"=w90:errorcluster, "MotorControlDeviceRef"=w89:T20)  [unwired: 7 in]
        n48 = call <vilib>:"Spark MAX Set Idle Mode.vi"("error in (no error)"=w90, "Idle Mode"=w88, "MotorControlDeviceRef in"=w89) -> ("error out"=w87:errorcluster, "MotorControlDeviceRef out"=w86:T20)  [unwired: 7 in]
        n49 = call <vilib>:"WPI_MotorControlRefNum Registry Set.vi"("error in (no error)"=w87, "refnum name"=w84, "MotorControlDevRef"=w86) -> ("error out"=w85:errorcluster)  [unwired: 7 in, 1 out]
      }
      n50 = in-place {
        in-place-border: w82 -> [w102]
        in-place-border: w81 -> [w101]
        w106 = TRUE  # Normally Closed
        n51 = Concatenate Strings(w101, "Count" ("refnum name")) -> (w99:string)
        n52 = Concatenate Strings(w99, "/" ("string"), "resetFLAG" ("string")) -> (w98:string)
        n53 = call-poly <vilib>:"WPI_SwitchOpen.vi"("Normally Closed"=w106, "error in (no error)"=w102, "DIO Channel"="KICKER COUNT DIO") -> ("error out"=w104:errorcluster, "SwitchDevRef"=w103:T28)  [unwired: 7 in]
        n54 = call <vilib>:"WPI_SwitchRefNum Registry Set.vi"("error in (no error)"=w104, "refnum name"=w99, "SwitchDevRef"=w103) -> ()  [unwired: 7 in, 2 out]
        n55 = call-poly <vilib>:"NT Write Value.vi"("Boolean"=TRUE, "Name"=w98) -> ()  [unwired: 9 in, 1 out]
      }
    }
  }
  n56 = in-place "LIFTING ARMS" {
    w108 = FALSE  # Invert climbers
    w109 = FALSE  # Invert arm actuators
    # "left & right screws - NEO brushless w/ Spark Max\nleft & right chain - Falcon 500\neach with limit switches (8 in all)"
    n57 = in-place {
      in-place-border: "FALCON Climbing config" -> [_]
      in-place-border: [w149] -> w112
      in-place-border: [w158] -> w111
      in-place-border: [w157] -> w110
      in-place-border: w109 -> [w152]
      in-place-border: w108 -> [w151]
      in-place-border: "Motor Control Neutral Mode" -> [w144]
      w157 = "ARM" ("refnum name")
      w158 = "Climber" ("refnum name")
      w156 = "LEFT" ("refnum name")
      # "LEFT"
      n58 = call <vilib>:"CTRE_Phoenix_TalonFX_Open.vi"("Invert"=w151, "Device Number"="CLIMBER LEFT CAN ID") -> ("error out"=w142:errorcluster, "PhoenixMotorControlDevRef"=w143:T20)  [unwired: 8 in]
      n59 = Concatenate Strings(w158, w156) -> (w153:string)
      n60 = call <vilib>:"CTRE_Phoenix_MotorControl_SetNeutralMode.vi"("error in (no error)"=w142, "Motor Control Neutral Mode"=w144, "PhoenixMotorControlDevRef"=w143) -> ("error out"=w146:errorcluster, "PhoenixMotorControlDevRef"=w145:T20)  [unwired: 7 in]
      n61 = call <vilib>:"CTRE_Phoenix_MotorControl_RefNumRegistrySet.vi"("error in (no error)"=w146, "refnum name"=w153, "PhoenixMotorControlDevRef"=w145) -> ("error out"=w155:errorcluster, "PhoenixMotorControlDevRef"=w154:T20)  [unwired: 7 in]
      n62 = call "WRITE Falcon500 values.vi"("PhoenixMotorControlDevRef"=w154, "refnum name"=w153, "error in (no error)"=w155) -> ()  [unwired: 5 in, 2 out]
      n63 = Concatenate Strings(w157, w156) -> (w147:string)
      n64 = call <vilib>:"Spark MAX Open.vi"("error in (no error)"=w155, "Invert"=w152, "Device Number"="ARM LEFT CAN ID") -> ("error out"=w160:errorcluster, "MotorControlDeviceRef"=w159:T20)  [unwired: 7 in]
      n65 = call <vilib>:"WPI_MotorControlRefNum Registry Set.vi"("error in (no error)"=w160, "refnum name"=w147, "MotorControlDevRef"=w159) -> ("error out"=w148:errorcluster, "MotorControlDevRef"=w150:T20)  [unwired: 7 in]
      n66 = call "CONFIG NEO ARM ACTUATORS.vi"("error in (no error)"=w148, "MotorControlDevRef"=w150, "RefName"=w147) -> ("error out"=w149:errorcluster)  [unwired: 8 in]
    }
    n67 = disable-structure shown="Disabled" {
      disable-tunnel: "FALCON Climbing config" -> [w120 _]
      disable-tunnel: w112 -> [w119 _]
      disable-tunnel: w111 -> [w118 _]
      disable-tunnel: w110 -> [w117 _]
      disable-tunnel: w109 -> [w116 _]
      disable-tunnel: w108 -> [w115 _]
      disable-tunnel: "Motor Control Neutral Mode" -> [w114 _]
      frame Disabled {
        n68 = in-place {
          in-place-border: w120 -> [_]
          in-place-border: w119 -> [w137]
          in-place-border: w118 -> [w136]
          in-place-border: w117 -> [w134]
          in-place-border: w116 -> [w131]
          in-place-border: w115 -> [w130]
          in-place-border: w114 -> [w126]
          w135 = "RIGHT" ("refnum name")
          # "RIGHT"
          n69 = call <vilib>:"CTRE_Phoenix_TalonFX_Open.vi"("Invert"=w130, "error in"=w137, "Device Number"="CLIMBER RIGHT CAN ID") -> ("error out"=w121:errorcluster, "PhoenixMotorControlDevRef"=w122:T20)  [unwired: 7 in]
          n70 = Concatenate Strings(w136, w135) -> (w132:string)
          n71 = call <vilib>:"CTRE_Phoenix_MotorControl_SetNeutralMode.vi"("error in (no error)"=w121, "Motor Control Neutral Mode"=w126, "PhoenixMotorControlDevRef"=w122) -> ("error out"=w124:errorcluster, "PhoenixMotorControlDevRef"=w123:T20)  [unwired: 7 in]
          n72 = Concatenate Strings(w134, w135) -> (w127:string)
          n73 = call <vilib>:"CTRE_Phoenix_MotorControl_RefNumRegistrySet.vi"("error in (no error)"=w124, "refnum name"=w132, "PhoenixMotorControlDevRef"=w123) -> ("error out"=w125:errorcluster, "PhoenixMotorControlDevRef"=w133:T20)  [unwired: 7 in]
          n74 = call <vilib>:"Spark MAX Open.vi"("error in (no error)"=w125, "Invert"=w131, "Device Number"="ARM RIGHT CAN ID") -> ("error out"=w139:errorcluster, "MotorControlDeviceRef"=w138:T20)  [unwired: 7 in]
          n75 = call "WRITE Falcon500 values.vi"("PhoenixMotorControlDevRef"=w133, "refnum name"=w132, "error in (no error)"=w125) -> ()  [unwired: 5 in, 2 out]
          n76 = call <vilib>:"WPI_MotorControlRefNum Registry Set.vi"("error in (no error)"=w139, "refnum name"=w127, "MotorControlDevRef"=w138) -> ("error out"=w128:errorcluster, "MotorControlDevRef"=w129:T20)  [unwired: 7 in]
          n77 = call "CONFIG NEO ARM ACTUATORS.vi"("error in (no error)"=w128, "MotorControlDevRef"=w129, "RefName"=w127) -> ()  [unwired: 8 in, 1 out]
        }
      }
      frame Enabled {
      }
    }
  }
  n78 = in-place "INPUT CONTROLS" {
    # "initialize a joystick"
    n79 = call <vilib>:"WPI_JoystickOpen.vi"("JoystickDevice"=WPI_JoystickDeviceEnum."USB 0") -> ("JoystickDevRef"=w164:T31)  [unwired: 10 in]
    n80 = call <vilib>:"WPI_JoystickRefNum Registry Set.vi"("refnum name"="Joystick 0", "JoystickDevRef"=w164) -> ()  [unwired: 8 in, 2 out]
  }
